vi "positive_waveform_sum.vi"(9 "plus-minus":bool[](array[boolean]), 11 "read in data":waveform(dbl)(graph) caption="waveform in") -> (2 "csapás impulzus":cluster{"Ramp Pattern":dbl[], dbl[]}(graph), 3 "Integral X":dbl[](array[numeric]))   [LabVIEW 2020]
uses:
  <vilib>/Analysis/1siggen.llb/Ramp Pattern by Samples.vi
  <vilib>/Waveform/WDTOps.llb/WDT Waveform to XY Pairs DBL.vi
  <vilib>/Analysis/NI_AALBase.lvlib
panel:
  out "inspection":cluster{timestamp[], dbl[]}[](graph)
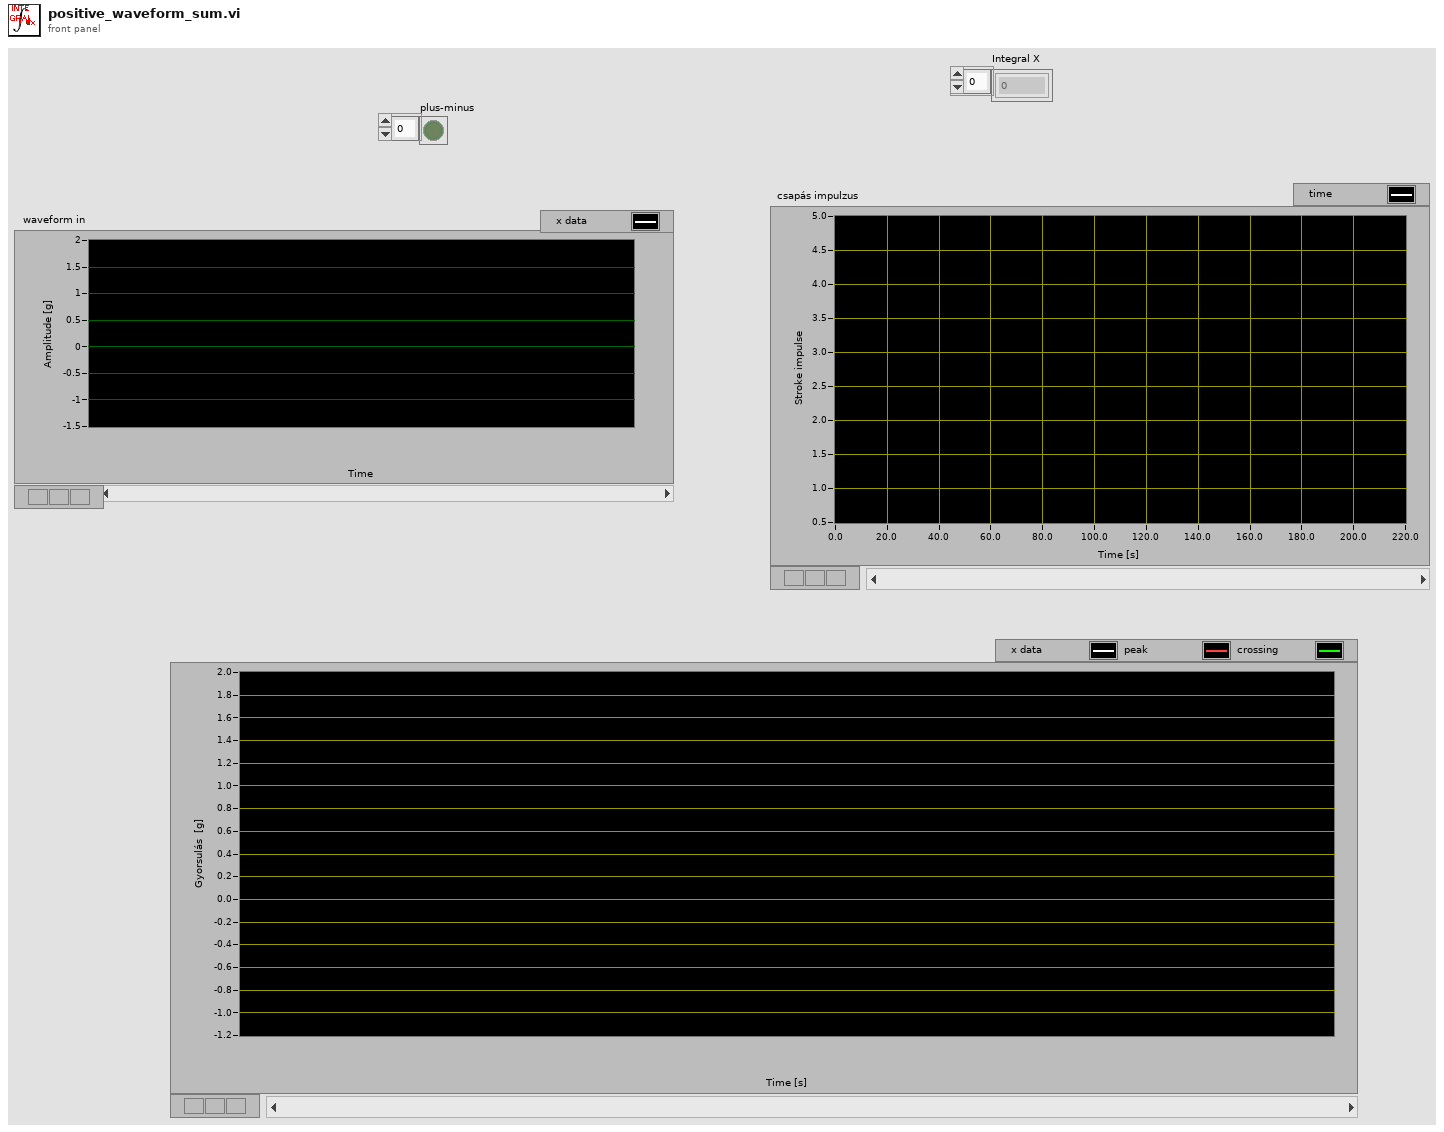
[diagram p1: front panel]
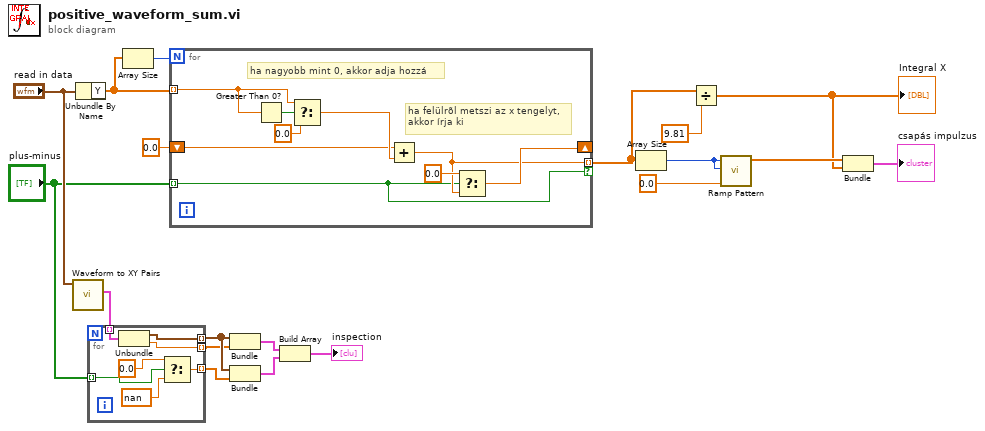
[diagram p0: block diagram]
diagram:
  n1 = call-poly <vilib>:"Waveform to XY Pairs.vi"("waveform in"="read in data") -> ("XY pairs"=w6:cluster{"x":timestamp, "y":dbl}[])  [unwired: 8 in, 2 out]
  n2 = Unbundle By Name("read in data") -> ("Y"=w15:dbl[])
  n3 = for {
    tunnel: "plus-minus" -> [w22] mode=indexing
    tunnel: [w23] -> w1 mode=indexing
    tunnel: w6 -> [w26] mode=indexing
    tunnel: [w25] -> w3 mode=indexing
    tunnel: [w24] -> w2 mode=indexing
    n4 = Unbundle(w26) -> ("x"=w25:timestamp, "y"=w24:dbl)
    n5 = Select(t=0.0, s=w22, f=nan) -> (s? t:f=w23:dbl)
  }
  n6 = Array Size(array=w15) -> (size(s)=w16:i32)
  n7 = for {
    N: w16 -> [_]
    tunnel: w15 -> [w35] mode=indexing
    shift-right: [w30] -> _
    shift-left: 0.0 -> [w31]
    tunnel: "plus-minus" -> [w27] mode=indexing
    tunnel: [w28] -> w10 mode=indexing if=w27
    # "ha felülrõl metszi az x tengelyt,\nakkor írja ki"
    # "ha nagyobb mint 0, akkor adja hozzá"
    n8 = Greater Than 0?(x=w35) -> (x > 0?=w32:bool)
    n9 = Select(t=w35, s=w32, f=0.0) -> (s? t:f=w33:dbl)
    n10 = Add(x=w31, y=w33) -> (x+y=w28:dbl)
    n11 = Select(t=0.0, s=w27, f=w28) -> (s? t:f=w30:dbl)
  }
  n12 = Bundle(w3, w2) -> (w4:cluster{timestamp[], dbl[]})  [unwired: 1 in]
  n13 = Bundle(w3, w1) -> (w5:cluster{timestamp[], dbl[]})  [unwired: 1 in]
  n14 = Build Array(w4, w5) -> (→"inspection":cluster{timestamp[], dbl[]}[])
  n15 = Array Size(array=w10) -> (size(s)=w18:i32)
  n16 = Divide(x=w10, y=9.81 ("x")) -> (x/y=w12:dbl[])
  "Integral X" <- w12
  n17 = call-poly <vilib>:"Ramp Pattern.vi"("start"=0.0, "end"=w18, "samples"=w18) -> ("Ramp Pattern"=w17:dbl[])  [unwired: 7 in, 1 out]
  n18 = Bundle("Ramp Pattern"=w17, w12) -> (→"csapás impulzus":cluster{"Ramp Pattern":dbl[], dbl[]})  [unwired: 1 in]
